vi "Wrap Text.vi"(10 "width":u32, 11 "item names":string[](array[string])) -> (2 "number of items wrapped":i32, 3 "item names with wrapping":string[](array[string]))   [LabVIEW 2021, in "CIF_UI.lvclass"]
doc: "This VI uses the <B>Get Nth Line</B> property to wrap text.\n\nDoug Norman"
uses:
  CIF_UI.lvclass
panel:
  out "width control":string
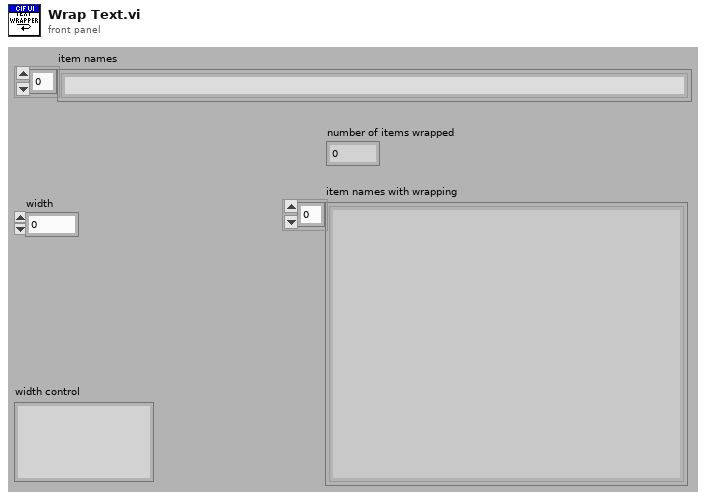
[diagram p1: front panel]
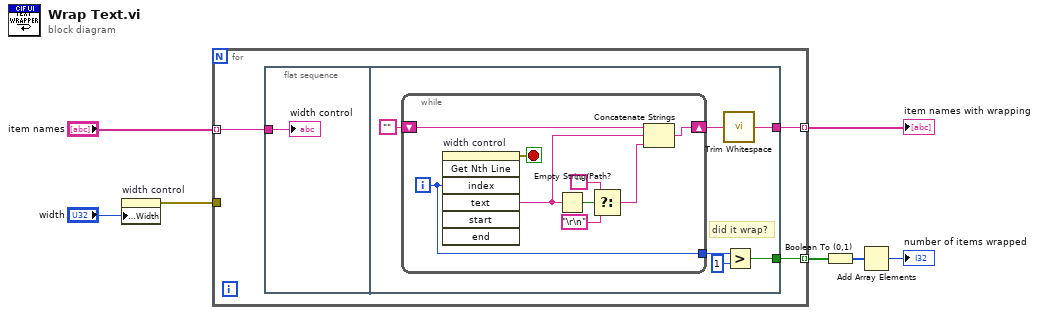
[diagram p0: block diagram]
diagram:
  n1 = property on="width control" class="Str"("Text Size:Width"="width") -> (error out=w1:errorcluster)  [unwired: 2 in, 1 out]
  n2 = for {
    tunnel: "item names" -> [w10] mode=indexing
    tunnel: [w9] -> w6 mode=indexing
    tunnel: [w8] -> w5 mode=indexing
    tunnel: w1 -> [_]
    n3 = flat-sequence {
      tunnel: w10 -> [w11]
      tunnel: [w15] -> w9
      tunnel: [w12] -> w8
      frame #0 {
        "width control" <- w11
      }
      frame #1 {
        # "did it wrap?"
        n4 = while {
          shift-right: [w18] -> w16
          shift-left: "" -> [w25]
          tunnel: [w19] -> w14
          i -> [w19]
          stop <- w26 stop-if-true
          n5 = invoke on="width control" class="Str" method="Get Nth Line"("index"=w19) -> (error out=w26:errorcluster, "text"=w21:string)  [unwired: 6 in, 5 out]
          n6 = Empty String/Path?(string/path=w21) -> (empty?=w22:bool)
          n7 = Select(t="", s=w22, f="\r\n") -> (s? t:f=w20:string)
          n8 = Concatenate Strings(w25, w21, w20) -> (w18:string)
        }
        n9 = call <vilib>:"Trim Whitespace.vi"("string"=w16) -> ("trimmed string"=w15:string)  [unwired: 1 in]
        n10 = Greater?(x=w14, y=1) -> (0:w12:bool)
      }
    }
  }
  "item names with wrapping" <- w6
  n11 = Boolean To (0,1)(Boolean=w5) -> (0, 1=w4:i16[])
  n12 = Add Array Elements(numeric array=w4) -> (sum=→"number of items wrapped":i16)
